vi "tampon.vi"() -> ()   [LabVIEW 2015]
panel:
  out "Curently at image:  2":string
  out "Curently at image:":string
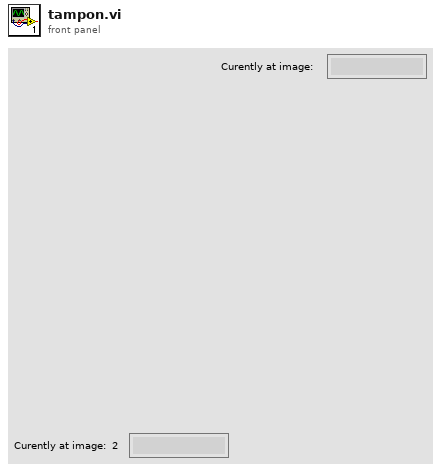
[diagram p1: front panel]
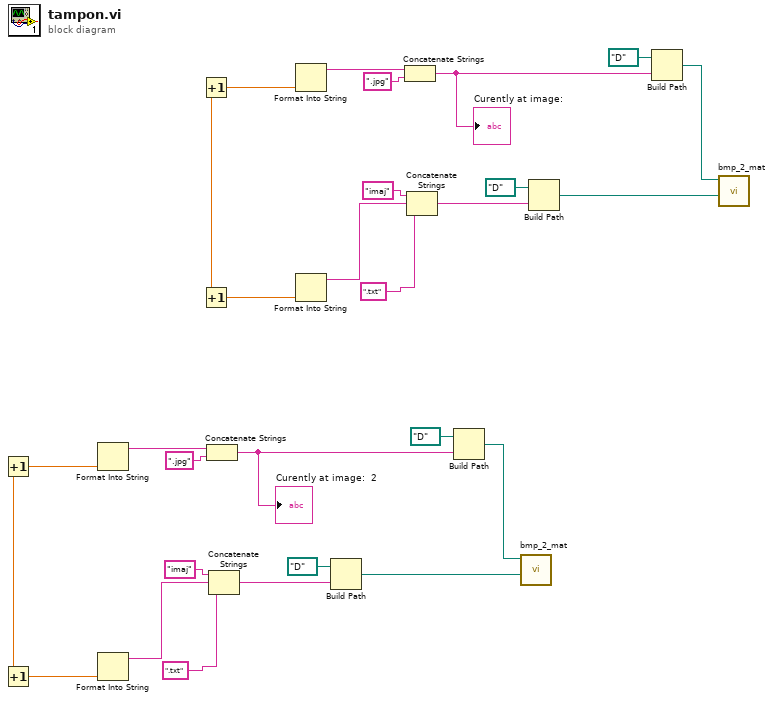
[diagram p0: block diagram]
diagram:
  n1 = Increment() -> (x=w1:dbl, x+1=w4:dbl)
  n2 = Increment(x=w1) -> (x+1=w5:dbl)
  n3 = Format Into String(w5) -> (resulting string=w13:string)  [unwired: 3 in, 1 out]
  n4 = Format Into String(w4) -> (resulting string=w10:string)  [unwired: 3 in, 1 out]
  n5 = Increment() -> (x=w17:dbl, x+1=w19:dbl)
  n6 = Increment(x=w17) -> (x+1=w18:dbl)
  n7 = Concatenate Strings(w13, ".jpg" ("string")) -> (w2:string)
  "Curently at image:  2" <- w2
  n8 = Concatenate Strings("imaj" ("string"), w10, ".txt" ("string")) -> (w7:string)
  n9 = Format Into String(w19) -> (resulting string=w27:string)  [unwired: 3 in, 1 out]
  n10 = Format Into String(w18) -> (resulting string=w24:string)  [unwired: 3 in, 1 out]
  n11 = Build Path(base path=path "D:/", name or relative path=w7) -> (appended path=w6:path)
  n12 = Concatenate Strings(w27, ".jpg" ("string")) -> (w15:string)
  "Curently at image:" <- w15
  n13 = Concatenate Strings("imaj" ("string"), w24, ".txt" ("string")) -> (w21:string)
  n14 = Build Path(base path=path "D:/", name or relative path=w2) -> (appended path=w3:path)
  n15 = call "bmp_2_mat.vi"("Destinatia1"=w6, "Imaginea1"=w3) -> ()  [unwired: 10 in]
  n16 = Build Path(base path=path "D:/", name or relative path=w21) -> (appended path=w20:path)
  n17 = Build Path(base path=path "D:/", name or relative path=w15) -> (appended path=w16:path)
  n18 = call "bmp_2_mat.vi"("Destinatia1"=w20, "Imaginea1"=w16) -> ()  [unwired: 10 in]
